vi "sub vi - Drive Relays All v6.vi"(9 "Array #2":bool[](array[boolean]), 10 "Array #1":bool[](array[boolean]), 11 "Array #0":bool[](array[boolean])) -> (0 "error Array":errorcluster[](array[cluster]))   [LabVIEW 2013]
panel:
  # "LAB01-1 (START)"
  # "LAB02-1 (JIG)"
  # "LAB04-2 (START)"
  # "LAB01-1 (JIG)"
  # "LAB03-1 (START)"
  # "LAB04-2 (JIG)"
  # "LAB01-2 (START)"
  # "LAB05-1 (START)"
  # "LAB03-1 (JIG)"
  # "LAB01-2 (JIG)"
  # "LAB05-1 (JIG)"
  # "LAB03-2 (START)"
  # "LAB02-1 (START)"
  # "LAB05-2 (START)"
  # "LAB03-2 (JIG)"
  # "LAB05-2 (JIG)"
  # "LAB02-1 (JIG)"
  # "LAB04-1 (START)"
  # "LAB02-1 (START)"
  # "LAB04-1 (JIG)"
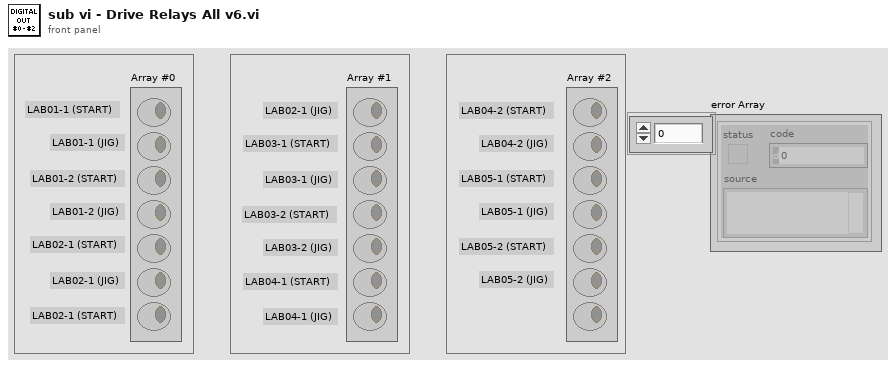
[diagram p1: front panel]
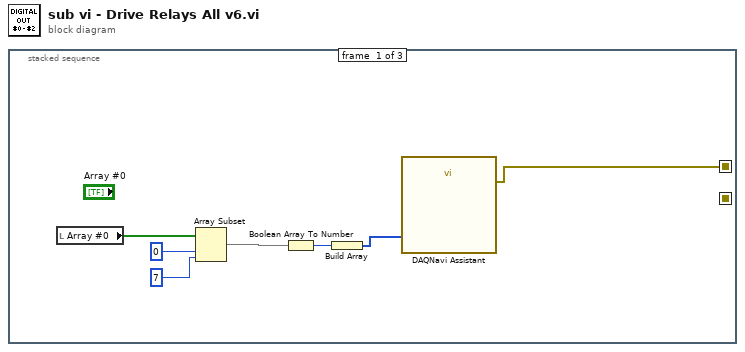
[diagram p0: block diagram]
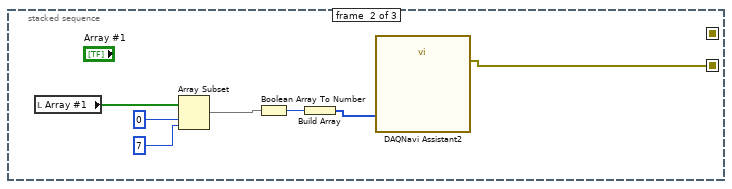
[diagram p2: hidden frame]
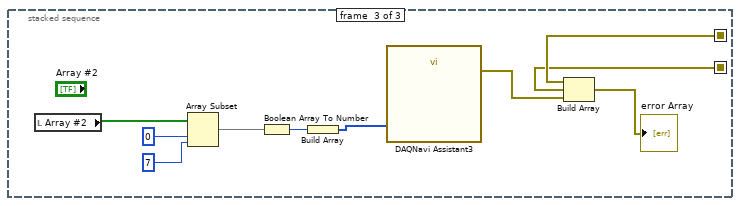
[diagram p3: hidden frame]
diagram:
  n1 = stacked-sequence {
    seq-local: [w1 _ _] -> [_ _ w18]
    seq-local: [_ w8 _] -> [_ _ w17]
    frame #0 {
      n2 = local read "Array #0"() -> (w5:bool[])
      n3 = Array Subset(array=w5, index=0, length=7) -> (w2:bool[])
      n4 = Boolean Array To Number(Boolean array=w2) -> (number=w7:u8)
      n5 = Build Array(w7) -> (w6:u8[])
      n6 = call "DAQNavi Assistant"("dataIn(U8Array)"=w6) -> ("error out"=w1:errorcluster)  [unwired: 26 in]
    }
    frame #1 {
      n7 = local read "Array #1"() -> (w10:bool[])
      n8 = Array Subset(array=w10, index=0, length=7) -> (w9:bool[])
      n9 = Boolean Array To Number(Boolean array=w9) -> (number=w14:u8)
      n10 = Build Array(w14) -> (w13:u8[])
      n11 = call "DAQNavi Assistant2"("dataIn(U8Array)"=w13) -> ("error out"=w8:errorcluster)  [unwired: 26 in]
    }
    frame #2 {
      n12 = local read "Array #2"() -> (w20:bool[])
      n13 = Array Subset(array=w20, index=0, length=7) -> (w19:bool[])
      n14 = Boolean Array To Number(Boolean array=w19) -> (number=w24:u8)
      n15 = Build Array(w24) -> (w23:u8[])
      n16 = call "DAQNavi Assistant3"("dataIn(U8Array)"=w23) -> ("error out"=w16:errorcluster)  [unwired: 26 in]
      n17 = Build Array(w18, w17, w16) -> (→"error Array":errorcluster[])
    }
  }
